vi "Write Header - CCD operation Mode.vi"(8 "error in (no error)":errorcluster, 11 "Save Image in":refnum<class "Save Image.lvclass">) -> (0 "error out":errorcluster, 3 "Save Image out":refnum<class "Save Image.lvclass">)   [LabVIEW 2018, in "Save Image.lvclass"]
uses:
  Save Image.lvclass
  Interface/Interface.lvclass
  <vilib>/Utility/Data Type/NI_Data Type.lvlib
  Simulated_Header/Simulated_Header.lvclass
  Simulated_Header/write keyword - string.vi
  Simulated_Header/write keyword - integer.vi
  Simulated_Header/write keyword - boolean.vi
  Simulated_Header/write keyword - float.vi
  <userlib>/atmcd32d.llb/AcquisitionMode_mode typedef.ctl
  <userlib>/atmcd32d.llb/ReadMode_mode typedef.ctl
  <userlib>/atmcd32d.llb/Shutter_mode typedef.ctl
panel:
  out "CCD Config":T4
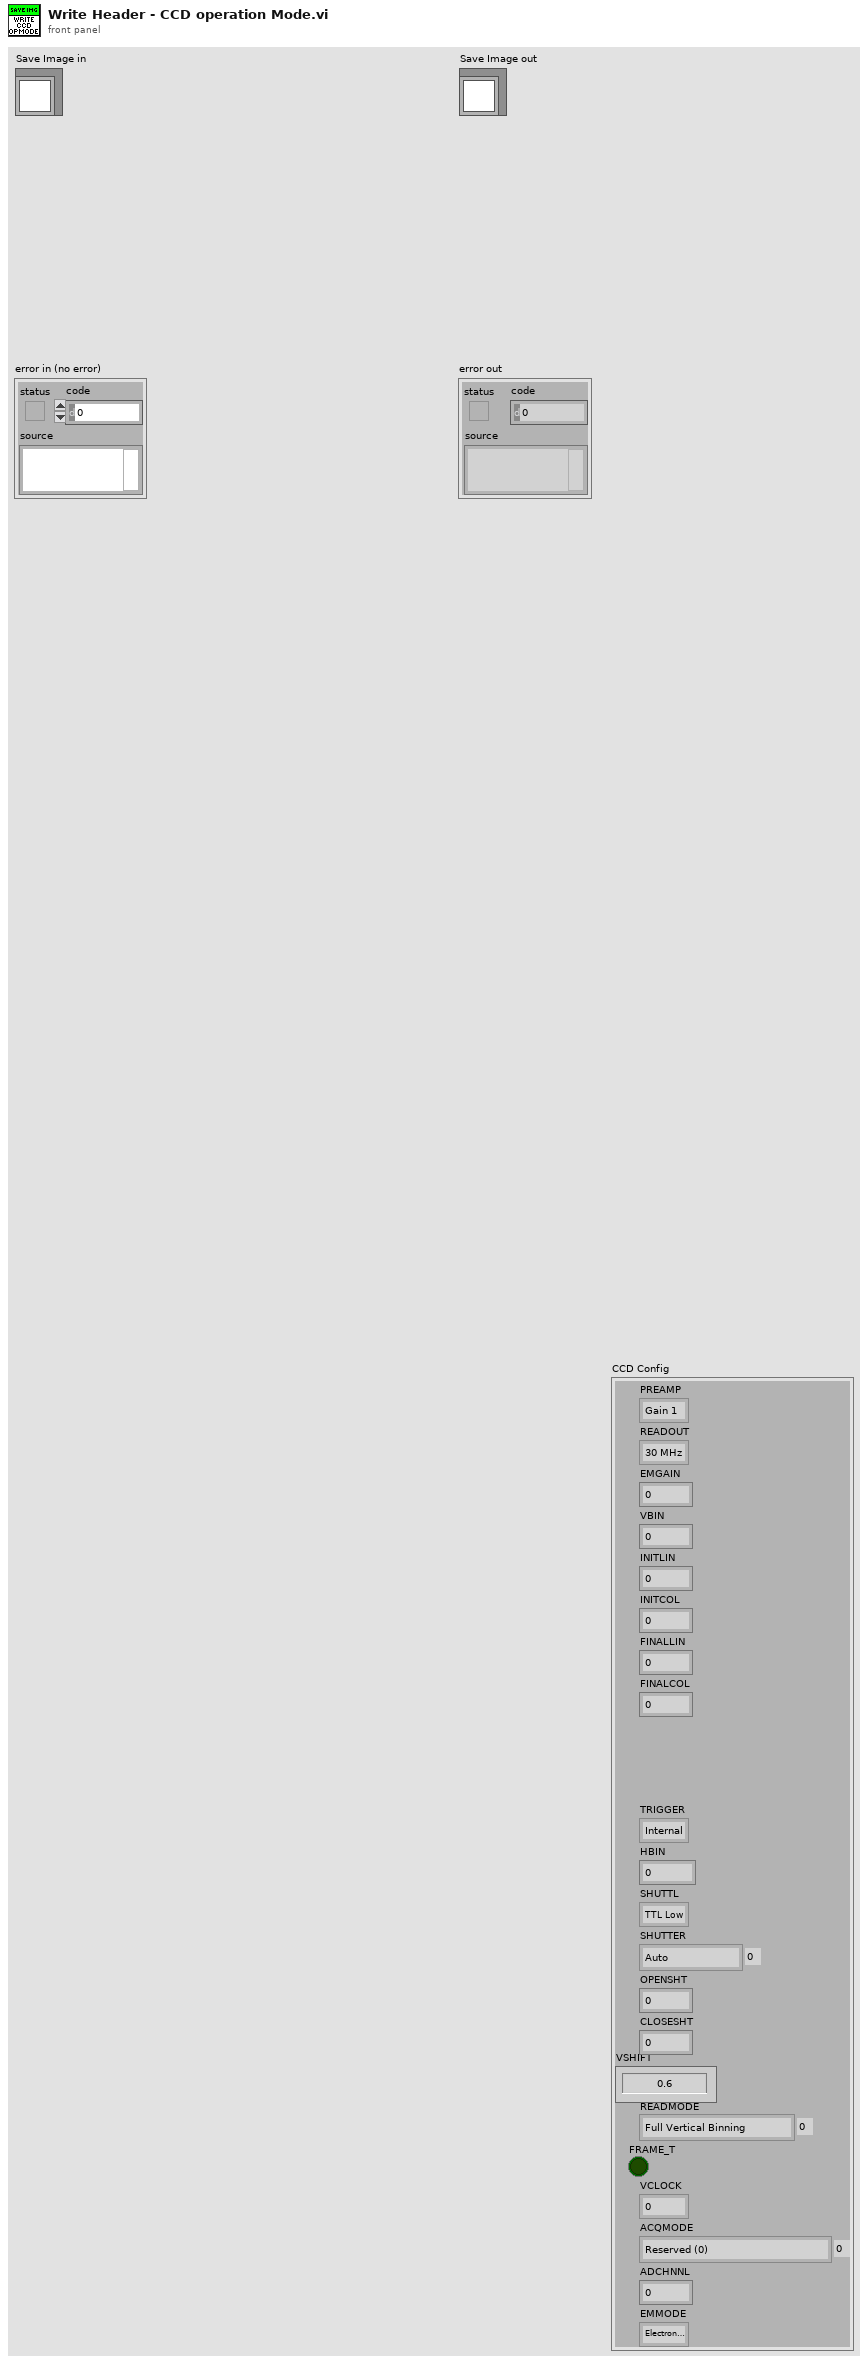
[diagram p1: front panel]
types:
  T1 = typedef "Shutter_mode typedef.ctl" = enum16{"Auto", "Open", "Close", "N/A (3)", "Open FVB Series", "Open Any Series"}
  T2 = typedef "ReadMode_mode typedef.ctl" = enum16{"Full Vertical Binning", "Multi-Track", "Random-Track", "Single-Track", "Image"}
  T3 = typedef "AcquisitionMode_mode typedef.ctl" = enum16{"Reserved (0)", "Single Scan", "Accumulate", "Kinetics", "Fast Kinetics", "Run Till Abort", "Reserved (6)", "Reserved (7)", "Reserved (8)", "Time Delayed Integration"}
  T4 = cluster{"PREAMP":enum16{"Gain 1", "Gain 2"}, "READOUT":enum16{"30 MHz", "20 MHz", "10 MHz", "1 MHz", "0.1 MHz"}, "EMGAIN":u16, "VBIN":u16, "INITLIN":u16, "INITCOL":u16, "FINALLIN":u16, "FINALCOL":u16, "TRIGGER":enum16{"Internal", "External", "N/A", "N/A_1", "N/A_2", "N/A_3", "External Start"}, "HBIN":u16, "SHUTTL":enum16{"TTL Low", "TTL High"}, "SHUTTER":T1, "OPENSHT":u16, "CLOSESHT":u16, "VSHIFT":enum16{"0.6", "1.13", "2.2", "4.33"}, "READMODE":T2, "FRAME_T":bool, "VCLOCK":enum16{"0", "+1", "+2", "+3", "+4"}, "ACQMODE":T3, "ADCHNNL":u16, "EMMODE":enum16{"Electron Multiplying", "Conventional"}}
  T5 = cluster{"PREAMP":u16, "READOUT_RATE":u16, "EM_GAIN":u16, "VBIN":u16, "INITIAL_LINE":u16, "INITIAL_COLUMN":u16, "FINAL_LINE":u16, "FINAL_COLUMN":u16, "TRIGGER_MODE":u16, "HBIN":u16, "SHUTTER_TTL":u16, "SHUTTER_MODE":u16, "SHUTTER_OPENING_TIME":u16, "SHUTTER_CLOSING_TIME":u16, "VERTICAL_SHIFT_SPEED":u16, "READ_MODE":u16, "FRAME_TRANSFER":bool, "VERTICAL_CLOCK_VOLTAGE":u16, "ACQUISITION_MODE":u16, "AD_CHANNEL":u16, "EM_MODE":u16}
  T6 = typedef "NI_Data Type.lvlib/Data Type.ctl" = enum8{"Invalid Type", "Void", "I8", "I16", "I32", "I64", "U8", "U16", "U32", "U64", "Single Float", "Double Float", "Extended Float", "Single Complex", "Double Complex", "Extended Complex", "Enum U8", "Enum U16", "Enum U32", "Enum U64", "Single Float With Unit", "Double Float With Unit", "Extended Float With Unit", "Single Complex with Unit", "Double Complex with Unit", "Extended Complex with Unit", "Boolean", "String", "Path", "Picture", "Tag", "Array", "Cluster", "Variant", "LV Variant", "Waveform", "Timestamp", "Digital Waveform", "Digital Data", "ExpressData", "Refnum", "External Data", "VI", "Poly VI", "LabVIEW Class Instance", "Fixed Point"}
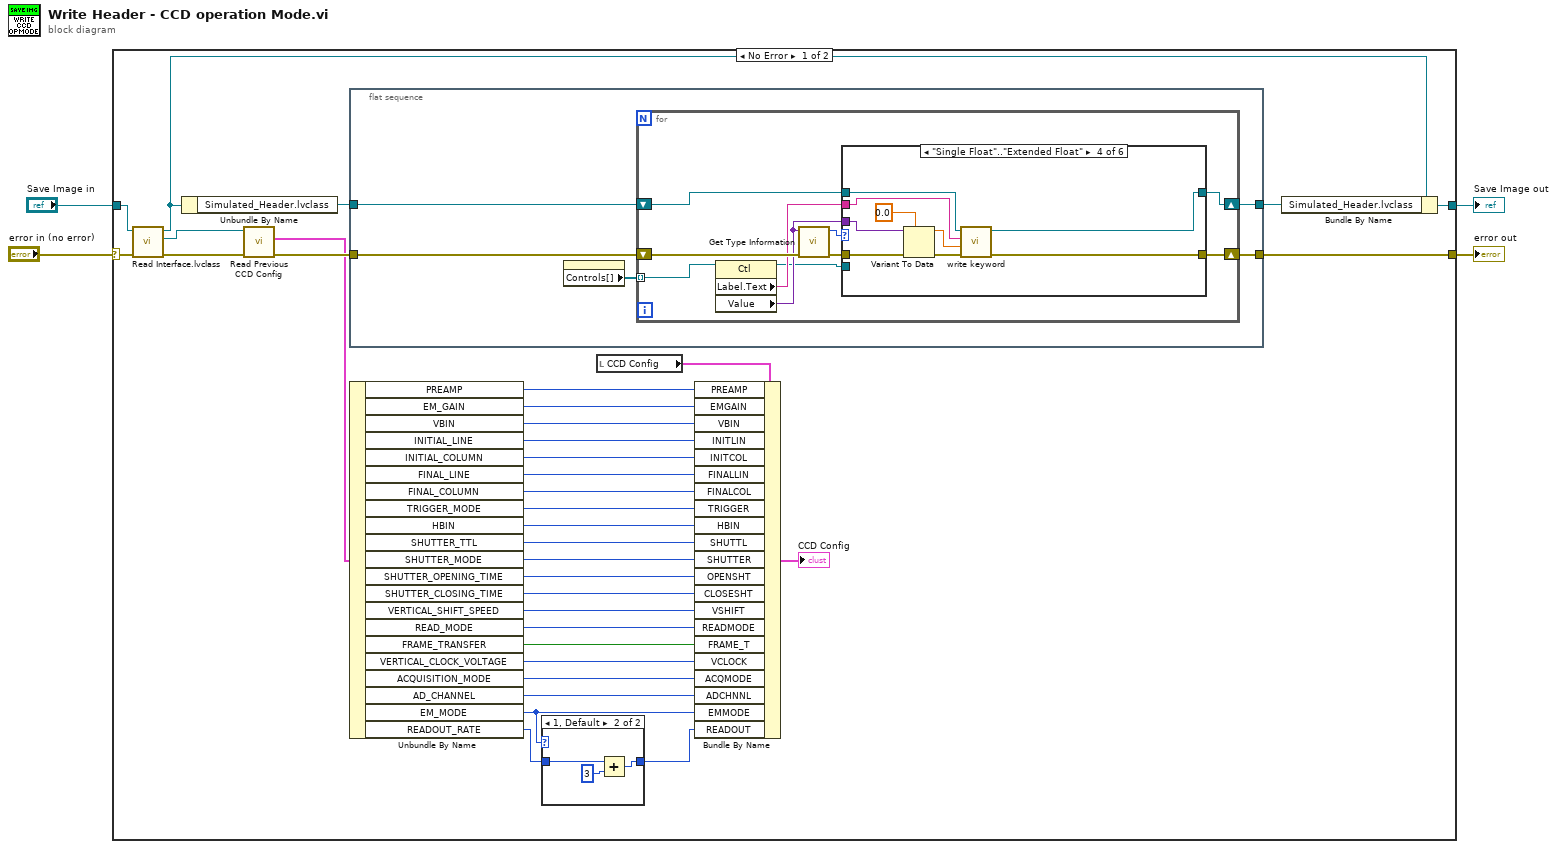
[diagram p0: block diagram]
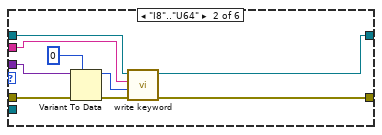
[diagram p4: hidden frame]
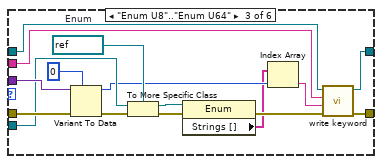
[diagram p5: hidden frame]
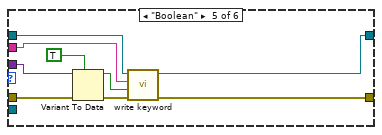
[diagram p6: hidden frame]
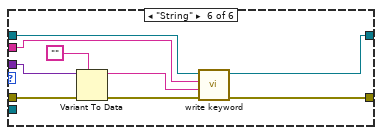
[diagram p7: hidden frame]
diagram:
  n1 = case shown="No Error" "error in (no error)" {
    selector: "error in (no error)" -> [w39 w113]
    tunnel: [w31 w113] -> w3
    tunnel: [w32 w114] -> w1
    tunnel: "Save Image in" -> [w38 w114]
    frame No Error {
      n2 = call "Read Interface.lvclass.vi"("error in (no error)"=w39, "Save Image in"=w38) -> ("error out"=w36:errorcluster, "Interface.lvclass"=w37:refnum<class "Interface.lvclass">, "Save Image out"=w35:refnum<class "Save Image.lvclass">)  [unwired: 7 in]
      n3 = Unbundle By Name(w35) -> ("Simulated_Header.lvclass"=w34:refnum<class "Simulated_Header.lvclass">)
      n4 = call "Read Previous CCD Config.vi"("error in (no error)"=w36, "Interface in"=w37) -> ("error out"=w33:errorcluster, "CCD Config"=w9:T5)  [unwired: 7 in, 1 out]
      n5 = flat-sequence {
        tunnel: [w48] -> w31
        tunnel: w34 -> [w47]
        tunnel: [w46] -> w5
        tunnel: w33 -> [w45]
        frame #0 {
          n6 = property on="CCD Config" class="Clust (strict)"() -> ("Controls[]"=w44:refnum<vi>[])  [unwired: 2 in, 2 out]
          n7 = for {
            shift-right: [w54] -> w46
            shift-left: w47 -> [w52]
            shift-right: [w55] -> w48
            shift-left: w45 -> [w58]
            tunnel: w44 -> [w51] mode=indexing
            n8 = property class="Ctl"(reference=w51) -> (reference out=w50:refnum<vi>, "Label.Text"=w56:string, "Value"=w53:variant)  [unwired: 1 in, 1 out]
            n9 = call <vilib>:"Get Type Information.vi"("error in (no error)"=w58, "Variant"=w53) -> ("error out"=w57:errorcluster, "Type"=w49:T6)  [unwired: 5 in, 3 out]
            n10 = case shown="\"Single Float\"..\"Extended Float\"" w49 {
              tunnel: w57 -> [w60 w69 w85 w94 w103 w112]
              tunnel: w56 -> [_ w65 w83 w90 w99 w108]
              tunnel: [w60 w64 w82 w89 w98 w107] -> w55
              tunnel: [w59 w63 w81 w88 w97 w106] -> w54
              tunnel: w53 -> [_ w62 w80 w87 w96 w105]
              tunnel: w52 -> [w59 w61 w79 w86 w95 w104]
              tunnel: w50 -> [_ _ w77 _ _ _]
              frame "Invalid Type", Default {
              }
              frame "I8".."U64" {
                n11 = Variant To Data(error in=w69, type=0, Variant=w62) -> (data=w66:i32, error out=w67:errorcluster)
                n12 = call-poly "write keyword.vi"("error in (no error)"=w67, "Value"=w66, "keyword"=w65, "Simulated_Header in"=w61) -> ("error out"=w64:errorcluster, "Simulated_Header out"=w63:refnum<class "Simulated_Header.lvclass">)  [unwired: 6 in]
              }
              frame "Enum U8".."Enum U64" {
                w73 = refnum<vi> refnum  # Enum
                n13 = Variant To Data(error in=w85, type=0, Variant=w80) -> (data=w72:i32, error out=w76:errorcluster)
                n14 = To More Specific Class(target class=w73, reference=w77, error in=w76) -> (specific class reference=w75:refnum<vi>, error out=w74:errorcluster)
                n15 = property on="Property Node" class="Enum"(reference=w75, error in=w74) -> (error out=w78:errorcluster, "Strings []"=w71:string[])  [unwired: 1 out]
                n16 = Index Array(array=w71, index=w72) -> (element=w70:string)
                n17 = call-poly "write keyword.vi"("error in (no error)"=w78, "value"=w70, "keyword"=w83, "Simulated_Header in"=w79) -> ("error out"=w82:errorcluster, "Simulated_Header out"=w81:refnum<class "Simulated_Header.lvclass">)  [unwired: 6 in]
              }
              frame "Single Float".."Extended Float" {
                n18 = Variant To Data(error in=w94, type=0.0, Variant=w87) -> (data=w91:dbl, error out=w92:errorcluster)
                n19 = call-poly "write keyword.vi"("error in (no error)"=w92, "Value"=w91, "keyword"=w90, "Simulated_Header in"=w86) -> ("error out"=w89:errorcluster, "Simulated_Header out"=w88:refnum<class "Simulated_Header.lvclass">)  [unwired: 6 in]
              }
              frame "Boolean" {
                n20 = Variant To Data(error in=w103, type=TRUE, Variant=w96) -> (data=w100:bool, error out=w101:errorcluster)
                n21 = call-poly "write keyword.vi"("error in (no error)"=w101, "value"=w100, "keyword"=w99, "Simulated_Header in"=w95) -> ("error out"=w98:errorcluster, "Simulated_Header out"=w97:refnum<class "Simulated_Header.lvclass">)  [unwired: 6 in]
              }
              frame "String" {
                n22 = Variant To Data(error in=w112, type="", Variant=w105) -> (data=w109:string, error out=w110:errorcluster)
                n23 = call-poly "write keyword.vi"("error in (no error)"=w110, "value"=w109, "keyword"=w108, "Simulated_Header in"=w104) -> ("error out"=w107:errorcluster, "Simulated_Header out"=w106:refnum<class "Simulated_Header.lvclass">)  [unwired: 6 in]
              }
            }
          }
        }
      }
      n24 = Unbundle By Name(w9) -> ("PREAMP"=w10:u16, "EM_GAIN"=w11:u16, "VBIN"=w12:u16, "INITIAL_LINE"=w13:u16, "INITIAL_COLUMN"=w14:u16, "FINAL_LINE"=w15:u16, "FINAL_COLUMN"=w16:u16, "TRIGGER_MODE"=w17:u16, "HBIN"=w18:u16, "SHUTTER_TTL"=w19:u16, "SHUTTER_MODE"=w20:u16, "SHUTTER_OPENING_TIME"=w21:u16, "SHUTTER_CLOSING_TIME"=w22:u16, "VERTICAL_SHIFT_SPEED"=w23:u16, "READ_MODE"=w24:u16, "FRAME_TRANSFER"=w25:bool, "VERTICAL_CLOCK_VOLTAGE"=w26:u16, "ACQUISITION_MODE"=w27:u16, "AD_CHANNEL"=w28:u16, "EM_MODE"=w8:u16, "READOUT_RATE"=w7:u16)
      n25 = case shown="1, Default" w8 {
        tunnel: w7 -> [w40 w43]
        tunnel: [w40 w41] -> w6
        frame 0 {
        }
        frame 1, Default {
          n26 = Add(x=w43, y=u16 3) -> (x+y=w41:u16)
        }
      }
      n27 = local read "CCD Config"() -> (w29:T4)
      n28 = Bundle By Name(cluster=w29, "PREAMP"=w10, "EMGAIN"=w11, "VBIN"=w12, "INITLIN"=w13, "INITCOL"=w14, "FINALLIN"=w15, "FINALCOL"=w16, "TRIGGER"=w17, "HBIN"=w18, "SHUTTL"=w19, "SHUTTER"=w20, "OPENSHT"=w21, "CLOSESHT"=w22, "VSHIFT"=w23, "READMODE"=w24, "FRAME_T"=w25, "VCLOCK"=w26, "ACQMODE"=w27, "ADCHNNL"=w28, "EMMODE"=w8, "READOUT"=w6) -> (→"CCD Config":T4)
      n29 = Bundle By Name(cluster=w35, "Simulated_Header.lvclass"=w5) -> (w32:refnum<class "Save Image.lvclass">)
    }
    frame Error {
    }
  }
  "error out" <- w3
  "Save Image out" <- w1
